vi "Multiarea SC.vi"() -> ()   [LabVIEW 2019]
doc: "This VI captures the region of the screen and displays it on the front panel continuously.\nCan be used to develop remote desktop applications."
uses:
  <vilib>/Utility/miscctls.llb/LVBoundsTypeDef.ctl
  System.Drawing
  <vilib>/Utility/inputDevices.llb/mouseAcquire.vi
  <vilib>/Utility/inputDevices.llb/closeMouse.vi
  <vilib>/wsapi/NI_WebServices.lvlib
panel:
  in  "Height2 (px)":i32=100
  in  "Width2 (px)":i32=600
  in  "Y offset":i32
  in  "X offset":i32=100
  out "Bar":picture
  in  "Height1 (px)":i32=60
  in  "Width1 (px)":i32=150
  out "Space":picture
  in  "stop":bool
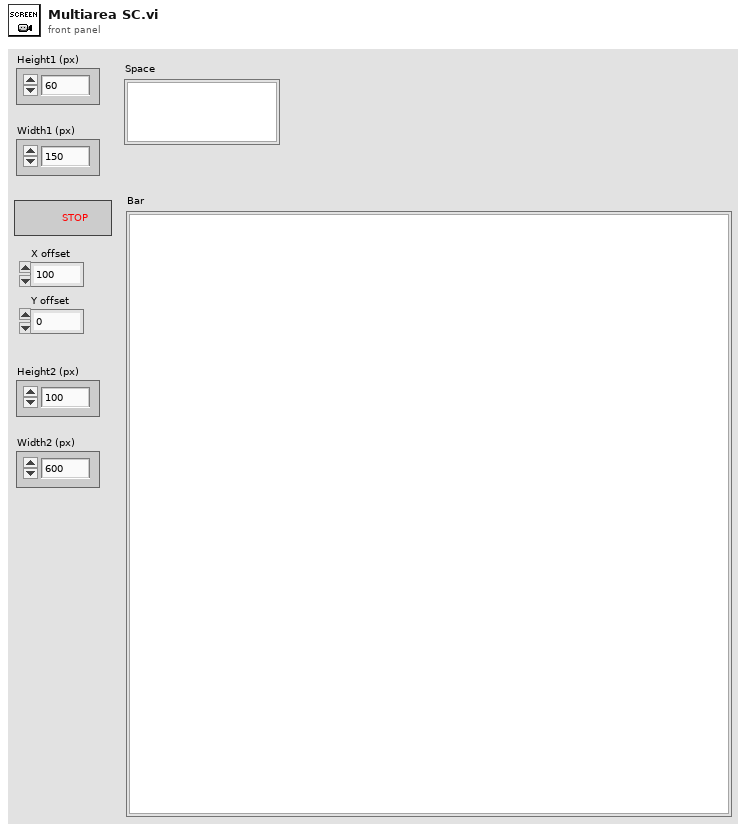
[diagram p1: front panel]
types:
  T1 = typedef "LVBoundsTypeDef.ctl" = cluster{"Width":u32, "Height":u32}
  T2 = cluster{"Horizontal":i32, "Vertical":i32, "Scrolling":i32}
  T3 = typedef "imagedata.ctl" = cluster{"image type":i32, "image depth":i32, "image":u8[], "mask":u8[], "colors":u32[], "Rectangle":cluster{"left":i16, "top":i16, "right":i16, "bottom":i16}}
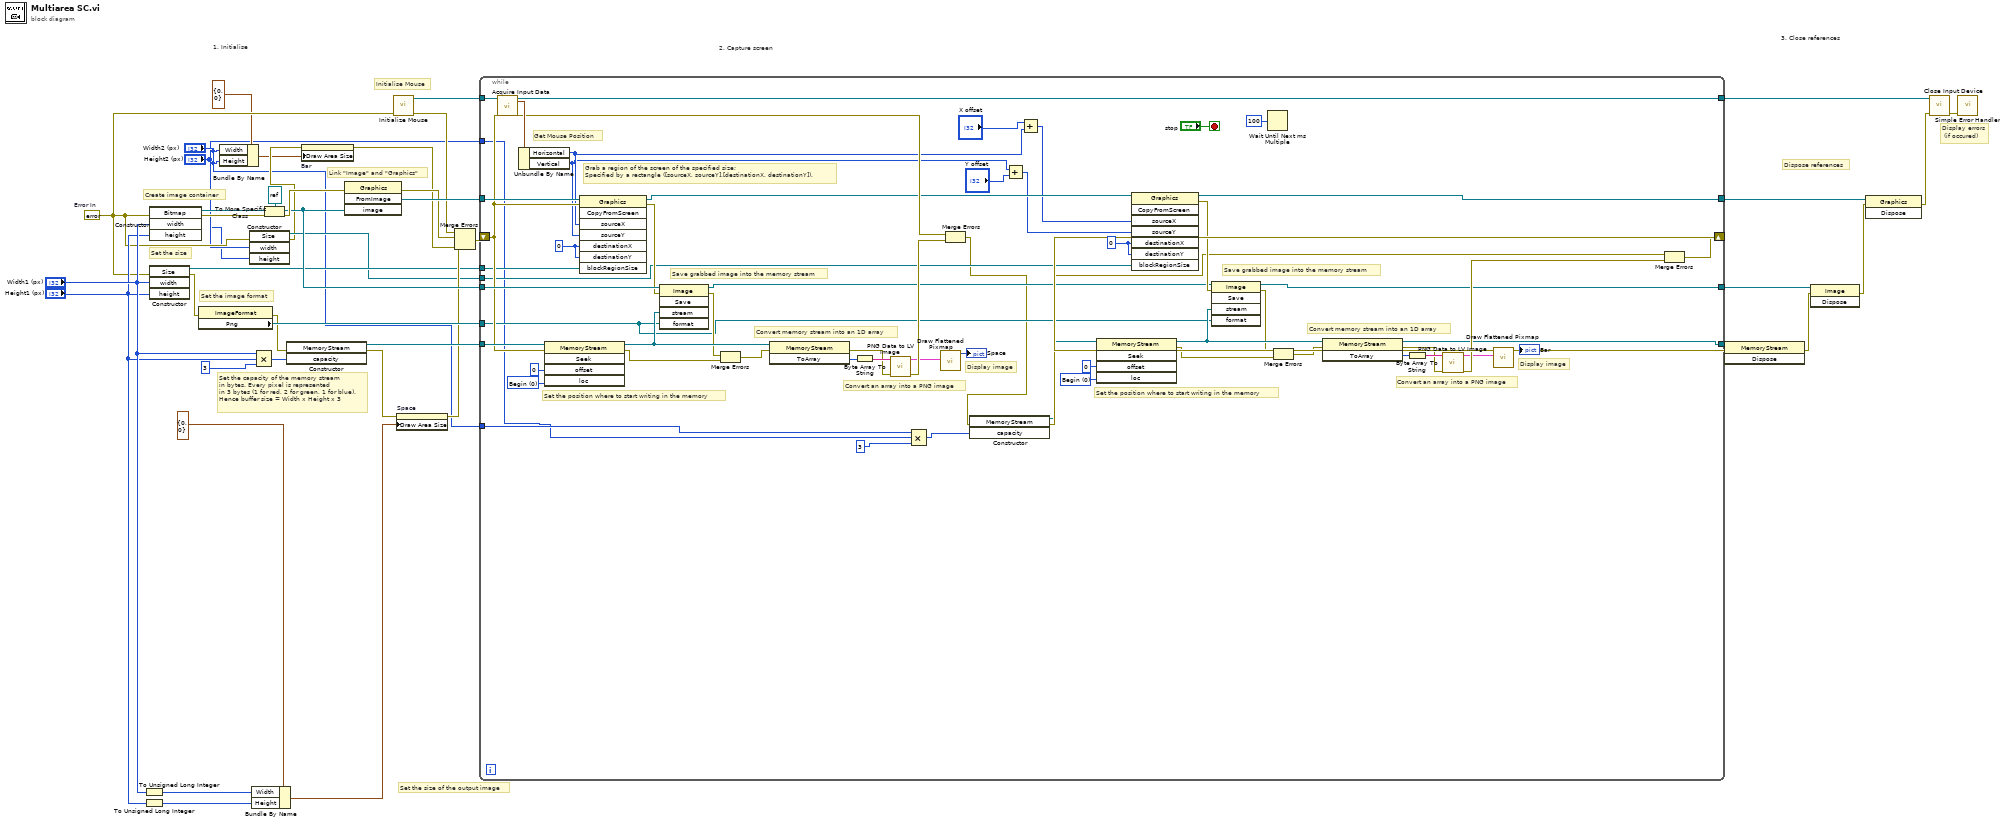
[diagram p0: block diagram]
diagram:
  w8 = errorcluster {"status"=FALSE, "code"=0, "source"=""}  # Error In
  # "Link \"Image\" and \"Graphics\""
  # "Set the size"
  # "Create image container"
  # "3. Close references"
  # "2. Capture screen"
  # "1. Initialise"
  # "Display errors\n (if occured)"
  # "Dispose references"
  # "Set the image format"
  # "Set the size of the output image"
  # "Set the capacity of the memory stream\nin bytes. Every pixel is represented\nin 3 bytes (1 for red, 2 for green, 1 for blue).\nHence buffer size = Width x Height x 3"
  # "Initialise Mouse"
  n1 = To Unsigned Long Integer(number="Width1 (px)") -> (unsigned 32bit integer=w17:u32)
  n2 = To Unsigned Long Integer(number="Height1 (px)") -> (unsigned 32bit integer=w15:u32)
  n3 = constructor class="Bitmap"(error in=w8, "width"="Width1 (px)", "height"="Height1 (px)") -> (reference out=w36:refnum<k24>, error out=w39:errorcluster)  [unwired: 2 in, 3 out]
  n4 = constructor class="Size"(error in=w8, "width"="Width1 (px)", "height"="Height1 (px)") -> (reference out=w9:refnum<k24>, error out=w26:errorcluster)  [unwired: 2 in, 3 out]
  n5 = property class="ImageFormat"(error in=w26) -> (error out=w25:errorcluster, "Png"=w34:refnum<k24>)  [unwired: 1 in, 1 out]
  n6 = Bundle By Name(cluster=T1 {"Width"=0, "Height"=0} ("Draw Area Size"), "Width"="Width2 (px)", "Height"="Width2 (px)") -> (w4:T1)
  n7 = constructor class="Size"(error in=w8, "width"="Width2 (px)", "height"="Height2 (px)") -> (reference out=w7:refnum<k24>, error out=w6:errorcluster)  [unwired: 2 in, 3 out]
  n8 = Bundle By Name(cluster=T1 {"Width"=0, "Height"=0} ("Draw Area Size"), "Width"=w17, "Height"=w15) -> (w21:T1)
  n9 = Compound Arithmetic op=MULTIPLY("Width1 (px)", "Height1 (px)", 3 ("value")) -> (w29:i32)
  n10 = To More Specific Class(target class=refnum<k24> refnum, reference=w36, error in=w39) -> (specific class reference=w28:refnum<k24>, error out=w40:errorcluster)
  n11 = constructor class="MemoryStream"(error in=w25, "capacity"=w29) -> (reference out=w31:refnum<k24>, error out=w20:errorcluster)  [unwired: 2 in, 2 out]
  n12 = property on="Bar" class="Pict"(error in=w6, "Draw Area Size"=w4) -> (error out=w5:errorcluster)  [unwired: 1 in, 1 out]
  n13 = invoke class="Graphics" method="FromImage"(error in=w40, "image"=w28) -> (error out=w24:errorcluster, "FromImage"=w37:refnum<k24>)  [unwired: 2 in, 2 out]
  n14 = call <vilib>:"Initialize Mouse.vi"("error in (no error)"=w8) -> ("error out"=w22:errorcluster, "device ID"=w42:refnum<k1>)  [unwired: 9 in]
  n15 = property on="Space" class="Pict"(error in=w20, "Draw Area Size"=w21) -> (error out=w19:errorcluster)  [unwired: 1 in, 1 out]
  n16 = Merge Errors(w22, w24, w19, w5) -> (w23:errorcluster)
  n17 = while {
    tunnel: w42 -> [w102]
    tunnel: [w100] -> w41
    tunnel: w37 -> [w99]
    tunnel: [w64] -> w35
    tunnel: w9 -> [w53]
    tunnel: w34 -> [w52]
    tunnel: [w62] -> w33
    tunnel: w31 -> [w96]
    tunnel: w28 -> [w89]
    shift-right: [w51] -> w14
    shift-left: w23 -> [w83]
    tunnel: [w60] -> w13
    tunnel: w7 -> [w50]
    tunnel: "Width2 (px)" -> [w45]
    tunnel: "Height2 (px)" -> [w44]
    stop <- "stop" stop-if-true
    w72 = 0 ("destinationX")
    w75 = 0 items=["Begin", "Current", "End"] ("loc")
    w90 = 0 ("destinationX")
    w94 = 0 items=["Begin", "Current", "End"] ("loc")
    # "Display image"
    # "Convert an array into a PNG image"
    # "Set the position where to start writing in the memory"
    # "Convert memory stream into an 1D array"
    # "Save grabbed image into the memory stream"
    # "Display image"
    # "Convert an array into a PNG image"
    # "Set the position where to start writing in the memory"
    # "Convert memory stream into an 1D array"
    # "Save grabbed image into the memory stream"
    # "Grab a region of the screen of the specified size;\nSpecified by a rectangle ([sourceX, sourceY],[destinationX, destinationY])."
    # "Get Mouse Position"
    n18 = call-poly <vilib>:"Acquire Input Data.vi"("device ID"=w102, "error in (no error)"=w83) -> ("device ID"=w100:refnum<k1>, "axis info"=w101:T2, "error out"=w82:errorcluster)  [unwired: 14 in, 1 out]
    n19 = Unbundle By Name(w101) -> ("Horizontal"=w59:i32, "Vertical"=w55:i32)
    n20 = invoke class="MemoryStream" method="Seek"(reference=w96, error in=w83, "offset"=i64 0, "loc"=w94) -> (reference out=w91:refnum<k24>, error out=w86:errorcluster)  [unwired: 1 in, 3 out]
    n21 = invoke class="Graphics" method="CopyFromScreen"(reference=w99, error in=w83, "sourceX"=w59, "sourceY"=w55, "destinationX"=w90, "destinationY"=w90, "blockRegionSize"=w53) -> (reference out=w61:refnum<k24>, error out=w84:errorcluster)  [unwired: 1 in, 6 out]
    n22 = invoke class="Image" method="Save"(reference=w89, error in=w84, "stream"=w91, "format"=w52) -> (reference out=w63:refnum<k24>, error out=w87:errorcluster)  [unwired: 1 in, 3 out]
    n23 = Merge Errors(w87, w86) -> (w85:errorcluster)
    n24 = invoke class="MemoryStream" method="ToArray"(reference=w91, error in=w85) -> (error out=w88:errorcluster, "ToArray"=w98:u8[])  [unwired: 1 in, 1 out]
    n25 = Byte Array To String(unsigned byte array=w98) -> (string=w97:string)
    n26 = call <vilib>:"PNG Data to LV Image.vi"("error in (no error)"=w88, "png data"=w97) -> ("error out"=w81:errorcluster, "image data"=w80:T3)  [unwired: 8 in]
    n27 = Compound Arithmetic op=MULTIPLY(w45, w44, 3 ("value")) -> (w46:i32)
    n28 = call <vilib>:"Draw Flattened Pixmap.vi"("image data"=w80) -> ("new picture"=→"Space":picture)  [unwired: 8 in]
    n29 = Merge Errors(w82, w81) -> (w49:errorcluster)
    n30 = constructor class="MemoryStream"(error in=w49, "capacity"=w46) -> (reference out=w43:refnum<k24>, error out=w48:errorcluster)  [unwired: 2 in, 2 out]
    n31 = Add(x=w55, y="Y offset") -> (x+y=w54:i32)
    n32 = Add(x="X offset", y=w59) -> (x+y=w58:i32)
    n33 = invoke class="MemoryStream" method="Seek"(reference=w43, "offset"=i64 0, "loc"=w75) -> (reference out=w73:refnum<k24>, error out=w69:errorcluster)  [unwired: 2 in, 3 out]
    n34 = invoke class="Graphics" method="CopyFromScreen"(reference=w61, "sourceX"=w58, "sourceY"=w54, "destinationX"=w72, "destinationY"=w72, "blockRegionSize"=w50) -> (reference out=w60:refnum<k24>, error out=w67:errorcluster)  [unwired: 2 in, 6 out]
    n35 = invoke class="Image" method="Save"(reference=w63, error in=w67, "stream"=w73, "format"=w52) -> (reference out=w62:refnum<k24>, error out=w70:errorcluster)  [unwired: 1 in, 3 out]
    n36 = Wait Until Next ms Multiple(millisecond multiple=u32 100) -> ()  [unwired: 1 out]
    n37 = Merge Errors(w70, w69) -> (w68:errorcluster)
    n38 = invoke class="MemoryStream" method="ToArray"(reference=w73, error in=w68) -> (reference out=w64:refnum<k24>, error out=w71:errorcluster, "ToArray"=w78:u8[])  [unwired: 1 in]
    n39 = Byte Array To String(unsigned byte array=w78) -> (string=w77:string)
    n40 = call <vilib>:"PNG Data to LV Image.vi"("error in (no error)"=w71, "png data"=w77) -> ("error out"=w66:errorcluster, "image data"=w65:T3)  [unwired: 8 in]
    n41 = call <vilib>:"Draw Flattened Pixmap.vi"("image data"=w65) -> ("new picture"=→"Bar":picture)  [unwired: 8 in]
    n42 = Merge Errors(w48, w66) -> (w51:errorcluster)
  }
  n43 = invoke class="MemoryStream" method="Dispose"(reference=w35, error in=w14) -> (error out=w32:errorcluster)  [unwired: 1 in, 2 out]
  n44 = invoke class="Image" method="Dispose"(reference=w33, error in=w32) -> (error out=w12:errorcluster)  [unwired: 1 in, 2 out]
  n45 = invoke class="Graphics" method="Dispose"(reference=w13, error in=w12) -> (error out=w11:errorcluster)  [unwired: 1 in, 2 out]
  n46 = call-poly <vilib>:"Close Input Device.vi"("error in (no error)"=w11, "device ID"=w41) -> ("error out"=w10:errorcluster)  [unwired: 8 in]
  n47 = call <vilib>:"Simple Error Handler.vi"("error in (no error)"=w10) -> ()  [unwired: 4 in, 5 out]
